vi "main(Test DQMH modules).vi"() -> ()   [LabVIEW 2018, in "Application.lvlib"] (continued)
      frame "Test DRV 27" {
        w4669 = 27  # DUT index(0-59)
        n2023 = disable-structure shown="LOGGING==TRUE" {
          disable-tunnel: w4670 -> [w4705 _]
          frame condition #0 (active) {
            n2024 = Empty String/Path?(string/path=w4705) -> (empty?=w4708:bool)
            n2025 = Select(t="Quece timeout", s=w4708, f=w4705) -> (s? t:f=w4704:string)
            n2026 = call "string log (SubVI).vi"("Enum"=enum16{"Init", "Log", "Read"}."Log", "state Name"=w4704) -> ()  [unwired: 8 in, 2 out]
          }
          frame condition #1 {
          }
        }
        n2027 = call "progress string(SubVI).vi"("String 3"=w4670, "String in"=w4671) -> ("String out"=w4672:string)  [unwired: 9 in]
        n2028 = call "FGV Driver Data.vi"("DUT index(1-60)"=w4669) -> ("DUT SC"=w4668:bool)  [unwired: 7 in, 3 out]
        n2029 = case shown="False" w4668 {
          tunnel: [w4697 _] -> w4677
          tunnel: w4674 -> [w4696 _]
          frame False {
            w4684 = T11 {"command"="", "command data"=variant} ("element")
            w4683 = "MEAS.mux6_1"
            n2030 = To Variant(anything=T4."mux6-1_channel0" ("mux6_1(3wires)_encode")) -> (Variant=w4682:variant)
            n2031 = To Variant(anything=T4."mux6_1_channel3_3" ("mux6_1(3wires)_encode")) -> (Variant=w4694:variant)
            n2032 = To Variant(anything=T4."mux6_1_channel3_2" ("mux6_1(3wires)_encode")) -> (Variant=w4692:variant)
            n2033 = Bundle By Name(cluster=w4684, "command"=w4683, "command data"=w4692) -> (w4691:T11)
            n2034 = Bundle By Name(cluster=w4684, "command"=w4683, "command data"=w4694) -> (w4690:T11)
            n2035 = Bundle By Name(cluster=w4684, "command"=w4683, "command data"=w4682) -> ()  [unwired: 1 out]
            n2036 = Bundle By Name(cluster=w4684, "command"="MEAS.DMM dual read") -> (w4688:T11)
            n2037 = Build Array(w4691, w4690, w4688) -> (w4686:T11[])
            n2038 = Reverse 1D Array(array=w4686) -> (reversed array=w4687:T11[])
            n2039 = for {
              tunnel: [w4703] -> w4697 mode=indexing
              tunnel: w4696 -> [w4702]
              tunnel: w4687 -> [w4701] mode=indexing
              n2040 = Unbundle By Name(w4701) -> ("command"=w4700:string, "command data"=w4699:variant)
              n2041 = call "App enquece.vi"("Priority Enquece"=TRUE, "command data"=w4699, "command"=w4700, "queue in"=w4702) -> ("error out"=w4703:errorcluster)  [unwired: 6 in, 1 out]
            }
          }
          frame True {
          }
        }
        n2042 = Merge Errors(w4675, w4677) -> (w4676:errorcluster)
      }
      frame "Test DRV 28" {
        w4710 = 28  # DUT index(0-59)
        n2043 = disable-structure shown="LOGGING==TRUE" {
          disable-tunnel: w4711 -> [w4746 _]
          frame condition #0 (active) {
            n2044 = Empty String/Path?(string/path=w4746) -> (empty?=w4749:bool)
            n2045 = Select(t="Quece timeout", s=w4749, f=w4746) -> (s? t:f=w4745:string)
            n2046 = call "string log (SubVI).vi"("Enum"=enum16{"Init", "Log", "Read"}."Log", "state Name"=w4745) -> ()  [unwired: 8 in, 2 out]
          }
          frame condition #1 {
          }
        }
        n2047 = call "progress string(SubVI).vi"("String 3"=w4711, "String in"=w4712) -> ("String out"=w4713:string)  [unwired: 9 in]
        n2048 = call "FGV Driver Data.vi"("DUT index(1-60)"=w4710) -> ("DUT SC"=w4709:bool)  [unwired: 7 in, 3 out]
        n2049 = case shown="False" w4709 {
          tunnel: [w4738 _] -> w4718
          tunnel: w4715 -> [w4737 _]
          frame False {
            w4723 = T11 {"command"="", "command data"=variant} ("element")
            w4725 = "MEAS.mux6_1"
            n2050 = To Variant(anything=T4."mux6-1_channel0" ("mux6_1(3wires)_encode")) -> (Variant=w4724:variant)
            n2051 = To Variant(anything=T4."mux6_1_channel4_3" ("mux6_1(3wires)_encode")) -> (Variant=w4735:variant)
            n2052 = To Variant(anything=T4."mux6_1_channel4_2" ("mux6_1(3wires)_encode")) -> (Variant=w4733:variant)
            n2053 = Bundle By Name(cluster=w4723, "command"=w4725, "command data"=w4733) -> (w4732:T11)
            n2054 = Bundle By Name(cluster=w4723, "command"=w4725, "command data"=w4735) -> (w4731:T11)
            n2055 = Bundle By Name(cluster=w4723, "command"=w4725, "command data"=w4724) -> ()  [unwired: 1 out]
            n2056 = Bundle By Name(cluster=w4723, "command"="MEAS.DMM dual read") -> (w4729:T11)
            n2057 = Build Array(w4732, w4731, w4729) -> (w4727:T11[])
            n2058 = Reverse 1D Array(array=w4727) -> (reversed array=w4728:T11[])
            n2059 = for {
              tunnel: [w4744] -> w4738 mode=indexing
              tunnel: w4737 -> [w4743]
              tunnel: w4728 -> [w4742] mode=indexing
              n2060 = Unbundle By Name(w4742) -> ("command"=w4741:string, "command data"=w4740:variant)
              n2061 = call "App enquece.vi"("Priority Enquece"=TRUE, "command data"=w4740, "command"=w4741, "queue in"=w4743) -> ("error out"=w4744:errorcluster)  [unwired: 6 in, 1 out]
            }
          }
          frame True {
          }
        }
        n2062 = Merge Errors(w4716, w4718) -> (w4717:errorcluster)
      }
      frame "Test DRV 29" {
        w4751 = 29  # DUT index(0-59)
        n2063 = disable-structure shown="LOGGING==TRUE" {
          disable-tunnel: w4752 -> [w4787 _]
          frame condition #0 (active) {
            n2064 = Empty String/Path?(string/path=w4787) -> (empty?=w4790:bool)
            n2065 = Select(t="Quece timeout", s=w4790, f=w4787) -> (s? t:f=w4786:string)
            n2066 = call "string log (SubVI).vi"("Enum"=enum16{"Init", "Log", "Read"}."Log", "state Name"=w4786) -> ()  [unwired: 8 in, 2 out]
          }
          frame condition #1 {
          }
        }
        n2067 = call "progress string(SubVI).vi"("String 3"=w4752, "String in"=w4753) -> ("String out"=w4754:string)  [unwired: 9 in]
        n2068 = call "FGV Driver Data.vi"("DUT index(1-60)"=w4751) -> ("DUT SC"=w4750:bool)  [unwired: 7 in, 3 out]
        n2069 = case shown="False" w4750 {
          tunnel: [w4779 _] -> w4759
          tunnel: w4756 -> [w4778 _]
          frame False {
            w4766 = T11 {"command"="", "command data"=variant} ("element")
            w4765 = "MEAS.mux6_1"
            n2070 = To Variant(anything=T4."mux6-1_channel0" ("mux6_1(3wires)_encode")) -> (Variant=w4764:variant)
            n2071 = To Variant(anything=T4."mux6_1_channel5_3" ("mux6_1(3wires)_encode")) -> (Variant=w4776:variant)
            n2072 = To Variant(anything=T4."mux6_1_channel5_2" ("mux6_1(3wires)_encode")) -> (Variant=w4774:variant)
            n2073 = Bundle By Name(cluster=w4766, "command"=w4765, "command data"=w4774) -> (w4773:T11)
            n2074 = Bundle By Name(cluster=w4766, "command"=w4765, "command data"=w4776) -> (w4772:T11)
            n2075 = Bundle By Name(cluster=w4766, "command"=w4765, "command data"=w4764) -> ()  [unwired: 1 out]
            n2076 = Bundle By Name(cluster=w4766, "command"="MEAS.DMM dual read") -> (w4770:T11)
            n2077 = Build Array(w4773, w4772, w4770) -> (w4768:T11[])
            n2078 = Reverse 1D Array(array=w4768) -> (reversed array=w4769:T11[])
            n2079 = for {
              tunnel: [w4785] -> w4779 mode=indexing
              tunnel: w4778 -> [w4784]
              tunnel: w4769 -> [w4783] mode=indexing
              n2080 = Unbundle By Name(w4783) -> ("command"=w4782:string, "command data"=w4781:variant)
              n2081 = call "App enquece.vi"("Priority Enquece"=TRUE, "command data"=w4781, "command"=w4782, "queue in"=w4784) -> ("error out"=w4785:errorcluster)  [unwired: 6 in, 1 out]
            }
          }
          frame True {
          }
        }
        n2082 = Merge Errors(w4757, w4759) -> (w4758:errorcluster)
      }
      frame "Test DRV 30" {
        w4791 = 30  # DUT index(0-59)
        n2083 = disable-structure shown="LOGGING==TRUE" {
          disable-tunnel: w4793 -> [w4828 _]
          frame condition #0 (active) {
            n2084 = Empty String/Path?(string/path=w4828) -> (empty?=w4831:bool)
            n2085 = Select(t="Quece timeout", s=w4831, f=w4828) -> (s? t:f=w4827:string)
            n2086 = call "string log (SubVI).vi"("Enum"=enum16{"Init", "Log", "Read"}."Log", "state Name"=w4827) -> ()  [unwired: 8 in, 2 out]
          }
          frame condition #1 {
          }
        }
        n2087 = call "progress string(SubVI).vi"("String 3"=w4793, "String in"=w4794) -> ("String out"=w4795:string)  [unwired: 9 in]
        n2088 = call "FGV Driver Data.vi"("DUT index(1-60)"=w4791) -> ("DUT SC"=w4792:bool)  [unwired: 7 in, 3 out]
        n2089 = case shown="False" w4792 {
          tunnel: [w4820 _] -> w4800
          tunnel: w4797 -> [w4819 _]
          frame False {
            w4807 = T11 {"command"="", "command data"=variant} ("element")
            w4806 = "MEAS.mux6_1"
            n2090 = To Variant(anything=T4."mux6-1_channel0" ("mux6_1(3wires)_encode")) -> (Variant=w4805:variant)
            n2091 = To Variant(anything=T4."mux6_1_channel6_3" ("mux6_1(3wires)_encode")) -> (Variant=w4817:variant)
            n2092 = To Variant(anything=T4."mux6_1_channel6_2" ("mux6_1(3wires)_encode")) -> (Variant=w4815:variant)
            n2093 = Bundle By Name(cluster=w4807, "command"=w4806, "command data"=w4815) -> (w4814:T11)
            n2094 = Bundle By Name(cluster=w4807, "command"=w4806, "command data"=w4817) -> (w4813:T11)
            n2095 = Bundle By Name(cluster=w4807, "command"=w4806, "command data"=w4805) -> ()  [unwired: 1 out]
            n2096 = Bundle By Name(cluster=w4807, "command"="MEAS.DMM dual read") -> (w4811:T11)
            n2097 = Build Array(w4814, w4813, w4811) -> (w4809:T11[])
            n2098 = Reverse 1D Array(array=w4809) -> (reversed array=w4810:T11[])
            n2099 = for {
              tunnel: [w4826] -> w4820 mode=indexing
              tunnel: w4819 -> [w4825]
              tunnel: w4810 -> [w4824] mode=indexing
              n2100 = Unbundle By Name(w4824) -> ("command"=w4823:string, "command data"=w4822:variant)
              n2101 = call "App enquece.vi"("Priority Enquece"=TRUE, "command data"=w4822, "command"=w4823, "queue in"=w4825) -> ("error out"=w4826:errorcluster)  [unwired: 6 in, 1 out]
            }
          }
          frame True {
          }
        }
        n2102 = Merge Errors(w4798, w4800) -> (w4799:errorcluster)
      }
      frame "Test DRV 31" {
        w4833 = 31  # DUT index(0-59)
        n2103 = disable-structure shown="LOGGING==TRUE" {
          disable-tunnel: w4834 -> [w4869 _]
          frame condition #0 (active) {
            n2104 = Empty String/Path?(string/path=w4869) -> (empty?=w4872:bool)
            n2105 = Select(t="Quece timeout", s=w4872, f=w4869) -> (s? t:f=w4868:string)
            n2106 = call "string log (SubVI).vi"("Enum"=enum16{"Init", "Log", "Read"}."Log", "state Name"=w4868) -> ()  [unwired: 8 in, 2 out]
          }
          frame condition #1 {
          }
        }
        n2107 = call "progress string(SubVI).vi"("String 3"=w4834, "String in"=w4835) -> ("String out"=w4836:string)  [unwired: 9 in]
        n2108 = call "FGV Driver Data.vi"("DUT index(1-60)"=w4833) -> ("DUT SC"=w4832:bool)  [unwired: 7 in, 3 out]
        n2109 = case shown="False" w4832 {
          tunnel: [w4861 _] -> w4841
          tunnel: w4838 -> [w4860 _]
          frame False {
            w4848 = T11 {"command"="", "command data"=variant} ("element")
            w4847 = "MEAS.mux6_1"
            n2110 = To Variant(anything=T4."mux6-1_channel0" ("mux6_1(3wires)_encode")) -> (Variant=w4846:variant)
            n2111 = To Variant(anything=T4."mux6_1_channel1_3" ("mux6_1(3wires)_encode")) -> (Variant=w4858:variant)
            n2112 = To Variant(anything=T4."mux6-1_channel1_2" ("mux6_1(3wires)_encode")) -> (Variant=w4856:variant)
            n2113 = Bundle By Name(cluster=w4848, "command"=w4847, "command data"=w4856) -> (w4855:T11)
            n2114 = Bundle By Name(cluster=w4848, "command"=w4847, "command data"=w4858) -> (w4854:T11)
            n2115 = Bundle By Name(cluster=w4848, "command"=w4847, "command data"=w4846) -> ()  [unwired: 1 out]
            n2116 = Bundle By Name(cluster=w4848, "command"="MEAS.DMM dual read") -> (w4852:T11)
            n2117 = Build Array(w4855, w4854, w4852) -> (w4850:T11[])
            n2118 = Reverse 1D Array(array=w4850) -> (reversed array=w4851:T11[])
            n2119 = for {
              tunnel: [w4867] -> w4861 mode=indexing
              tunnel: w4860 -> [w4866]
              tunnel: w4851 -> [w4865] mode=indexing
              n2120 = Unbundle By Name(w4865) -> ("command"=w4864:string, "command data"=w4863:variant)
              n2121 = call "App enquece.vi"("Priority Enquece"=TRUE, "command data"=w4863, "command"=w4864, "queue in"=w4866) -> ("error out"=w4867:errorcluster)  [unwired: 6 in, 1 out]
            }
          }
          frame True {
          }
        }
        n2122 = Merge Errors(w4839, w4841) -> (w4840:errorcluster)
      }
      frame "Test DRV 32" {
        w4874 = 32  # DUT index(0-59)
        n2123 = disable-structure shown="LOGGING==TRUE" {
          disable-tunnel: w4875 -> [w4910 _]
          frame condition #0 (active) {
            n2124 = Empty String/Path?(string/path=w4910) -> (empty?=w4913:bool)
            n2125 = Select(t="Quece timeout", s=w4913, f=w4910) -> (s? t:f=w4909:string)
            n2126 = call "string log (SubVI).vi"("Enum"=enum16{"Init", "Log", "Read"}."Log", "state Name"=w4909) -> ()  [unwired: 8 in, 2 out]
          }
          frame condition #1 {
          }
        }
        n2127 = call "progress string(SubVI).vi"("String 3"=w4875, "String in"=w4876) -> ("String out"=w4877:string)  [unwired: 9 in]
        n2128 = call "FGV Driver Data.vi"("DUT index(1-60)"=w4874) -> ("DUT SC"=w4873:bool)  [unwired: 7 in, 3 out]
        n2129 = case shown="False" w4873 {
          tunnel: [w4902 _] -> w4882
          tunnel: w4879 -> [w4901 _]
          frame False {
            w4889 = T11 {"command"="", "command data"=variant} ("element")
            w4888 = "MEAS.mux6_1"
            n2130 = To Variant(anything=T4."mux6-1_channel0" ("mux6_1(3wires)_encode")) -> (Variant=w4887:variant)
            n2131 = To Variant(anything=T4."mux6_1_channel2_3" ("mux6_1(3wires)_encode")) -> (Variant=w4899:variant)
            n2132 = To Variant(anything=T4."mux6_1_channel2_2" ("mux6_1(3wires)_encode")) -> (Variant=w4897:variant)
            n2133 = Bundle By Name(cluster=w4889, "command"=w4888, "command data"=w4897) -> (w4896:T11)
            n2134 = Bundle By Name(cluster=w4889, "command"=w4888, "command data"=w4899) -> (w4895:T11)
            n2135 = Bundle By Name(cluster=w4889, "command"=w4888, "command data"=w4887) -> ()  [unwired: 1 out]
            n2136 = Bundle By Name(cluster=w4889, "command"="MEAS.DMM dual read") -> (w4893:T11)
            n2137 = Build Array(w4896, w4895, w4893) -> (w4891:T11[])
            n2138 = Reverse 1D Array(array=w4891) -> (reversed array=w4892:T11[])
            n2139 = for {
              tunnel: [w4908] -> w4902 mode=indexing
              tunnel: w4901 -> [w4907]
              tunnel: w4892 -> [w4906] mode=indexing
              n2140 = Unbundle By Name(w4906) -> ("command"=w4905:string, "command data"=w4904:variant)
              n2141 = call "App enquece.vi"("Priority Enquece"=TRUE, "command data"=w4904, "command"=w4905, "queue in"=w4907) -> ("error out"=w4908:errorcluster)  [unwired: 6 in, 1 out]
            }
          }
          frame True {
          }
        }
        n2142 = Merge Errors(w4880, w4882) -> (w4881:errorcluster)
      }
      frame "Test DRV 33" {
        w4915 = 33  # DUT index(0-59)
        n2143 = disable-structure shown="LOGGING==TRUE" {
          disable-tunnel: w4916 -> [w4951 _]
          frame condition #0 (active) {
            n2144 = Empty String/Path?(string/path=w4951) -> (empty?=w4954:bool)
            n2145 = Select(t="Quece timeout", s=w4954, f=w4951) -> (s? t:f=w4950:string)
            n2146 = call "string log (SubVI).vi"("Enum"=enum16{"Init", "Log", "Read"}."Log", "state Name"=w4950) -> ()  [unwired: 8 in, 2 out]
          }
          frame condition #1 {
          }
        }
        n2147 = call "progress string(SubVI).vi"("String 3"=w4916, "String in"=w4917) -> ("String out"=w4918:string)  [unwired: 9 in]
        n2148 = call "FGV Driver Data.vi"("DUT index(1-60)"=w4915) -> ("DUT SC"=w4914:bool)  [unwired: 7 in, 3 out]
        n2149 = case shown="False" w4914 {
          tunnel: [w4943 _] -> w4923
          tunnel: w4920 -> [w4942 _]
          frame False {
            w4930 = T11 {"command"="", "command data"=variant} ("element")
            w4929 = "MEAS.mux6_1"
            n2150 = To Variant(anything=T4."mux6-1_channel0" ("mux6_1(3wires)_encode")) -> (Variant=w4928:variant)
            n2151 = To Variant(anything=T4."mux6_1_channel3_3" ("mux6_1(3wires)_encode")) -> (Variant=w4940:variant)
            n2152 = To Variant(anything=T4."mux6_1_channel3_2" ("mux6_1(3wires)_encode")) -> (Variant=w4938:variant)
            n2153 = Bundle By Name(cluster=w4930, "command"=w4929, "command data"=w4938) -> (w4937:T11)
            n2154 = Bundle By Name(cluster=w4930, "command"=w4929, "command data"=w4940) -> (w4936:T11)
            n2155 = Bundle By Name(cluster=w4930, "command"=w4929, "command data"=w4928) -> ()  [unwired: 1 out]
            n2156 = Bundle By Name(cluster=w4930, "command"="MEAS.DMM dual read") -> (w4934:T11)
            n2157 = Build Array(w4937, w4936, w4934) -> (w4932:T11[])
            n2158 = Reverse 1D Array(array=w4932) -> (reversed array=w4933:T11[])
            n2159 = for {
              tunnel: [w4949] -> w4943 mode=indexing
              tunnel: w4942 -> [w4948]
              tunnel: w4933 -> [w4947] mode=indexing
              n2160 = Unbundle By Name(w4947) -> ("command"=w4946:string, "command data"=w4945:variant)
              n2161 = call "App enquece.vi"("Priority Enquece"=TRUE, "command data"=w4945, "command"=w4946, "queue in"=w4948) -> ("error out"=w4949:errorcluster)  [unwired: 6 in, 1 out]
            }
          }
          frame True {
          }
        }
        n2162 = Merge Errors(w4921, w4923) -> (w4922:errorcluster)
      }
      frame "Test DRV 34" {
        w4956 = 34  # DUT index(0-59)
        n2163 = disable-structure shown="LOGGING==TRUE" {
          disable-tunnel: w4957 -> [w4992 _]
          frame condition #0 (active) {
            n2164 = Empty String/Path?(string/path=w4992) -> (empty?=w4995:bool)
            n2165 = Select(t="Quece timeout", s=w4995, f=w4992) -> (s? t:f=w4991:string)
            n2166 = call "string log (SubVI).vi"("Enum"=enum16{"Init", "Log", "Read"}."Log", "state Name"=w4991) -> ()  [unwired: 8 in, 2 out]
          }
          frame condition #1 {
          }
        }
        n2167 = call "progress string(SubVI).vi"("String 3"=w4957, "String in"=w4958) -> ("String out"=w4959:string)  [unwired: 9 in]
        n2168 = call "FGV Driver Data.vi"("DUT index(1-60)"=w4956) -> ("DUT SC"=w4955:bool)  [unwired: 7 in, 3 out]
        n2169 = case shown="False" w4955 {
          tunnel: [w4984 _] -> w4964
          tunnel: w4961 -> [w4983 _]
          frame False {
            w4971 = T11 {"command"="", "command data"=variant} ("element")
            w4970 = "MEAS.mux6_1"
            n2170 = To Variant(anything=T4."mux6-1_channel0" ("mux6_1(3wires)_encode")) -> (Variant=w4969:variant)
            n2171 = To Variant(anything=T4."mux6_1_channel4_3" ("mux6_1(3wires)_encode")) -> (Variant=w4981:variant)
            n2172 = To Variant(anything=T4."mux6_1_channel4_2" ("mux6_1(3wires)_encode")) -> (Variant=w4979:variant)
            n2173 = Bundle By Name(cluster=w4971, "command"=w4970, "command data"=w4979) -> (w4978:T11)
            n2174 = Bundle By Name(cluster=w4971, "command"=w4970, "command data"=w4981) -> (w4977:T11)
            n2175 = Bundle By Name(cluster=w4971, "command"=w4970, "command data"=w4969) -> ()  [unwired: 1 out]
            n2176 = Bundle By Name(cluster=w4971, "command"="MEAS.DMM dual read") -> (w4975:T11)
            n2177 = Build Array(w4978, w4977, w4975) -> (w4973:T11[])
            n2178 = Reverse 1D Array(array=w4973) -> (reversed array=w4974:T11[])
            n2179 = for {
              tunnel: [w4990] -> w4984 mode=indexing
              tunnel: w4983 -> [w4989]
              tunnel: w4974 -> [w4988] mode=indexing
              n2180 = Unbundle By Name(w4988) -> ("command"=w4987:string, "command data"=w4986:variant)
              n2181 = call "App enquece.vi"("Priority Enquece"=TRUE, "command data"=w4986, "command"=w4987, "queue in"=w4989) -> ("error out"=w4990:errorcluster)  [unwired: 6 in, 1 out]
            }
          }
          frame True {
          }
        }
        n2182 = Merge Errors(w4962, w4964) -> (w4963:errorcluster)
      }
      frame "Test DRV 35" {
        w4997 = 35  # DUT index(0-59)
        n2183 = disable-structure shown="LOGGING==TRUE" {
          disable-tunnel: w4998 -> [w5033 _]
          frame condition #0 (active) {
            n2184 = Empty String/Path?(string/path=w5033) -> (empty?=w5036:bool)
            n2185 = Select(t="Quece timeout", s=w5036, f=w5033) -> (s? t:f=w5032:string)
            n2186 = call "string log (SubVI).vi"("Enum"=enum16{"Init", "Log", "Read"}."Log", "state Name"=w5032) -> ()  [unwired: 8 in, 2 out]
          }
          frame condition #1 {
          }
        }
        n2187 = call "progress string(SubVI).vi"("String 3"=w4998, "String in"=w4999) -> ("String out"=w5000:string)  [unwired: 9 in]
        n2188 = call "FGV Driver Data.vi"("DUT index(1-60)"=w4997) -> ("DUT SC"=w4996:bool)  [unwired: 7 in, 3 out]
        n2189 = case shown="False" w4996 {
          tunnel: [w5025 _] -> w5005
          tunnel: w5002 -> [w5024 _]
          frame False {
            w5012 = T11 {"command"="", "command data"=variant} ("element")
            w5011 = "MEAS.mux6_1"
            n2190 = To Variant(anything=T4."mux6-1_channel0" ("mux6_1(3wires)_encode")) -> (Variant=w5010:variant)
            n2191 = To Variant(anything=T4."mux6_1_channel5_3" ("mux6_1(3wires)_encode")) -> (Variant=w5022:variant)
            n2192 = To Variant(anything=T4."mux6_1_channel5_2" ("mux6_1(3wires)_encode")) -> (Variant=w5020:variant)
            n2193 = Bundle By Name(cluster=w5012, "command"=w5011, "command data"=w5020) -> (w5019:T11)
            n2194 = Bundle By Name(cluster=w5012, "command"=w5011, "command data"=w5022) -> (w5018:T11)
            n2195 = Bundle By Name(cluster=w5012, "command"=w5011, "command data"=w5010) -> ()  [unwired: 1 out]
            n2196 = Bundle By Name(cluster=w5012, "command"="MEAS.DMM dual read") -> (w5016:T11)
            n2197 = Build Array(w5019, w5018, w5016) -> (w5014:T11[])
            n2198 = Reverse 1D Array(array=w5014) -> (reversed array=w5015:T11[])
            n2199 = for {
              tunnel: [w5031] -> w5025 mode=indexing
              tunnel: w5024 -> [w5030]
              tunnel: w5015 -> [w5029] mode=indexing
              n2200 = Unbundle By Name(w5029) -> ("command"=w5028:string, "command data"=w5027:variant)
              n2201 = call "App enquece.vi"("Priority Enquece"=TRUE, "command data"=w5027, "command"=w5028, "queue in"=w5030) -> ("error out"=w5031:errorcluster)  [unwired: 6 in, 1 out]
            }
          }
          frame True {
          }
        }
        n2202 = Merge Errors(w5003, w5005) -> (w5004:errorcluster)
      }
      frame "Test DRV 36" {
        w5038 = 36  # DUT index(0-59)
        n2203 = disable-structure shown="LOGGING==TRUE" {
          disable-tunnel: w5039 -> [w5074 _]
          frame condition #0 (active) {
            n2204 = Empty String/Path?(string/path=w5074) -> (empty?=w5077:bool)
            n2205 = Select(t="Quece timeout", s=w5077, f=w5074) -> (s? t:f=w5073:string)
            n2206 = call "string log (SubVI).vi"("Enum"=enum16{"Init", "Log", "Read"}."Log", "state Name"=w5073) -> ()  [unwired: 8 in, 2 out]
          }
          frame condition #1 {
          }
        }
        n2207 = call "progress string(SubVI).vi"("String 3"=w5039, "String in"=w5040) -> ("String out"=w5041:string)  [unwired: 9 in]
        n2208 = call "FGV Driver Data.vi"("DUT index(1-60)"=w5038) -> ("DUT SC"=w5037:bool)  [unwired: 7 in, 3 out]
        n2209 = case shown="False" w5037 {
          tunnel: [w5066 _] -> w5046
          tunnel: w5043 -> [w5065 _]
          frame False {
            w5053 = T11 {"command"="", "command data"=variant} ("element")
            w5052 = "MEAS.mux6_1"
            n2210 = To Variant(anything=T4."mux6-1_channel0" ("mux6_1(3wires)_encode")) -> (Variant=w5051:variant)
            n2211 = To Variant(anything=T4."mux6_1_channel6_3" ("mux6_1(3wires)_encode")) -> (Variant=w5063:variant)
            n2212 = To Variant(anything=T4."mux6_1_channel6_2" ("mux6_1(3wires)_encode")) -> (Variant=w5061:variant)
            n2213 = Bundle By Name(cluster=w5053, "command"=w5052, "command data"=w5061) -> (w5060:T11)
            n2214 = Bundle By Name(cluster=w5053, "command"=w5052, "command data"=w5063) -> (w5059:T11)
            n2215 = Bundle By Name(cluster=w5053, "command"=w5052, "command data"=w5051) -> ()  [unwired: 1 out]
            n2216 = Bundle By Name(cluster=w5053, "command"="MEAS.DMM dual read") -> (w5057:T11)
            n2217 = Build Array(w5060, w5059, w5057) -> (w5055:T11[])
            n2218 = Reverse 1D Array(array=w5055) -> (reversed array=w5056:T11[])
            n2219 = for {
              tunnel: [w5072] -> w5066 mode=indexing
              tunnel: w5065 -> [w5071]
              tunnel: w5056 -> [w5070] mode=indexing
              n2220 = Unbundle By Name(w5070) -> ("command"=w5069:string, "command data"=w5068:variant)
              n2221 = call "App enquece.vi"("Priority Enquece"=TRUE, "command data"=w5068, "command"=w5069, "queue in"=w5071) -> ("error out"=w5072:errorcluster)  [unwired: 6 in, 1 out]
            }
          }
          frame True {
          }
        }
        n2222 = Merge Errors(w5044, w5046) -> (w5045:errorcluster)
      }
      frame "Test DRV 37" {
        w5079 = 37  # DUT index(0-59)
        n2223 = disable-structure shown="LOGGING==TRUE" {
          disable-tunnel: w5080 -> [w5115 _]
          frame condition #0 (active) {
            n2224 = Empty String/Path?(string/path=w5115) -> (empty?=w5118:bool)
            n2225 = Select(t="Quece timeout", s=w5118, f=w5115) -> (s? t:f=w5114:string)
            n2226 = call "string log (SubVI).vi"("Enum"=enum16{"Init", "Log", "Read"}."Log", "state Name"=w5114) -> ()  [unwired: 8 in, 2 out]
          }
          frame condition #1 {
          }
        }
        n2227 = call "progress string(SubVI).vi"("String 3"=w5080, "String in"=w5081) -> ("String out"=w5082:string)  [unwired: 9 in]
        n2228 = call "FGV Driver Data.vi"("DUT index(1-60)"=w5079) -> ("DUT SC"=w5078:bool)  [unwired: 7 in, 3 out]
        n2229 = case shown="False" w5078 {
          tunnel: [w5107 _] -> w5087
          tunnel: w5084 -> [w5106 _]
          frame False {
            w5094 = T11 {"command"="", "command data"=variant} ("element")
            w5093 = "MEAS.mux6_1"
            n2230 = To Variant(anything=T4."mux6-1_channel0" ("mux6_1(3wires)_encode")) -> (Variant=w5092:variant)
            n2231 = To Variant(anything=T4."mux6_1_channel1_3" ("mux6_1(3wires)_encode")) -> (Variant=w5104:variant)
            n2232 = To Variant(anything=T4."mux6-1_channel1_2" ("mux6_1(3wires)_encode")) -> (Variant=w5102:variant)
            n2233 = Bundle By Name(cluster=w5094, "command"=w5093, "command data"=w5102) -> (w5101:T11)
            n2234 = Bundle By Name(cluster=w5094, "command"=w5093, "command data"=w5104) -> (w5100:T11)
            n2235 = Bundle By Name(cluster=w5094, "command"=w5093, "command data"=w5092) -> ()  [unwired: 1 out]
            n2236 = Bundle By Name(cluster=w5094, "command"="MEAS.DMM dual read") -> (w5098:T11)
            n2237 = Build Array(w5101, w5100, w5098) -> (w5096:T11[])
            n2238 = Reverse 1D Array(array=w5096) -> (reversed array=w5097:T11[])
            n2239 = for {
              tunnel: [w5113] -> w5107 mode=indexing
              tunnel: w5106 -> [w5112]
              tunnel: w5097 -> [w5111] mode=indexing
              n2240 = Unbundle By Name(w5111) -> ("command"=w5110:string, "command data"=w5109:variant)
              n2241 = call "App enquece.vi"("Priority Enquece"=TRUE, "command data"=w5109, "command"=w5110, "queue in"=w5112) -> ("error out"=w5113:errorcluster)  [unwired: 6 in, 1 out]
            }
          }
          frame True {
          }
        }
        n2242 = Merge Errors(w5085, w5087) -> (w5086:errorcluster)
      }
      frame "Test DRV 38" {
        w5120 = 38  # DUT index(0-59)
        n2243 = disable-structure shown="LOGGING==TRUE" {
          disable-tunnel: w5121 -> [w5156 _]
          frame condition #0 (active) {
            n2244 = Empty String/Path?(string/path=w5156) -> (empty?=w5159:bool)
            n2245 = Select(t="Quece timeout", s=w5159, f=w5156) -> (s? t:f=w5155:string)
            n2246 = call "string log (SubVI).vi"("Enum"=enum16{"Init", "Log", "Read"}."Log", "state Name"=w5155) -> ()  [unwired: 8 in, 2 out]
          }
          frame condition #1 {
          }
        }
        n2247 = call "progress string(SubVI).vi"("String 3"=w5121, "String in"=w5122) -> ("String out"=w5123:string)  [unwired: 9 in]
        n2248 = call "FGV Driver Data.vi"("DUT index(1-60)"=w5120) -> ("DUT SC"=w5119:bool)  [unwired: 7 in, 3 out]
        n2249 = case shown="False" w5119 {
          tunnel: [w5148 _] -> w5128
          tunnel: w5125 -> [w5147 _]
          frame False {
            w5135 = T11 {"command"="", "command data"=variant} ("element")
            w5134 = "MEAS.mux6_1"
            n2250 = To Variant(anything=T4."mux6-1_channel0" ("mux6_1(3wires)_encode")) -> (Variant=w5133:variant)
            n2251 = To Variant(anything=T4."mux6_1_channel2_3" ("mux6_1(3wires)_encode")) -> (Variant=w5145:variant)
            n2252 = To Variant(anything=T4."mux6_1_channel2_2" ("mux6_1(3wires)_encode")) -> (Variant=w5143:variant)
            n2253 = Bundle By Name(cluster=w5135, "command"=w5134, "command data"=w5143) -> (w5142:T11)
            n2254 = Bundle By Name(cluster=w5135, "command"=w5134, "command data"=w5145) -> (w5141:T11)
            n2255 = Bundle By Name(cluster=w5135, "command"=w5134, "command data"=w5133) -> ()  [unwired: 1 out]
            n2256 = Bundle By Name(cluster=w5135, "command"="MEAS.DMM dual read") -> (w5139:T11)
            n2257 = Build Array(w5142, w5141, w5139) -> (w5137:T11[])
            n2258 = Reverse 1D Array(array=w5137) -> (reversed array=w5138:T11[])
            n2259 = for {
              tunnel: [w5154] -> w5148 mode=indexing
              tunnel: w5147 -> [w5153]
              tunnel: w5138 -> [w5152] mode=indexing
              n2260 = Unbundle By Name(w5152) -> ("command"=w5151:string, "command data"=w5150:variant)
              n2261 = call "App enquece.vi"("Priority Enquece"=TRUE, "command data"=w5150, "command"=w5151, "queue in"=w5153) -> ("error out"=w5154:errorcluster)  [unwired: 6 in, 1 out]
            }
          }
          frame True {
          }
        }
        n2262 = Merge Errors(w5126, w5128) -> (w5127:errorcluster)
      }
      frame "Test DRV 39" {
        w5160 = 39  # DUT index(0-59)
        n2263 = disable-structure shown="LOGGING==TRUE" {
          disable-tunnel: w5162 -> [w5197 _]
          frame condition #0 (active) {
            n2264 = Empty String/Path?(string/path=w5197) -> (empty?=w5200:bool)
            n2265 = Select(t="Quece timeout", s=w5200, f=w5197) -> (s? t:f=w5196:string)
            n2266 = call "string log (SubVI).vi"("Enum"=enum16{"Init", "Log", "Read"}."Log", "state Name"=w5196) -> ()  [unwired: 8 in, 2 out]
          }
          frame condition #1 {
          }
        }
        n2267 = call "progress string(SubVI).vi"("String 3"=w5162, "String in"=w5163) -> ("String out"=w5164:string)  [unwired: 9 in]
        n2268 = call "FGV Driver Data.vi"("DUT index(1-60)"=w5160) -> ("DUT SC"=w5161:bool)  [unwired: 7 in, 3 out]
        n2269 = case shown="False" w5161 {
          tunnel: [w5189 _] -> w5169
          tunnel: w5166 -> [w5188 _]
          frame False {
            w5176 = T11 {"command"="", "command data"=variant} ("element")
            w5175 = "MEAS.mux6_1"
            n2270 = To Variant(anything=T4."mux6-1_channel0" ("mux6_1(3wires)_encode")) -> (Variant=w5174:variant)
            n2271 = To Variant(anything=T4."mux6_1_channel3_3" ("mux6_1(3wires)_encode")) -> (Variant=w5186:variant)
            n2272 = To Variant(anything=T4."mux6_1_channel3_2" ("mux6_1(3wires)_encode")) -> (Variant=w5184:variant)
            n2273 = Bundle By Name(cluster=w5176, "command"=w5175, "command data"=w5184) -> (w5183:T11)
            n2274 = Bundle By Name(cluster=w5176, "command"=w5175, "command data"=w5186) -> (w5182:T11)
            n2275 = Bundle By Name(cluster=w5176, "command"=w5175, "command data"=w5174) -> ()  [unwired: 1 out]
            n2276 = Bundle By Name(cluster=w5176, "command"="MEAS.DMM dual read") -> (w5180:T11)
            n2277 = Build Array(w5183, w5182, w5180) -> (w5178:T11[])
            n2278 = Reverse 1D Array(array=w5178) -> (reversed array=w5179:T11[])
            n2279 = for {
              tunnel: [w5195] -> w5189 mode=indexing
              tunnel: w5188 -> [w5194]
              tunnel: w5179 -> [w5193] mode=indexing
              n2280 = Unbundle By Name(w5193) -> ("command"=w5192:string, "command data"=w5191:variant)
              n2281 = call "App enquece.vi"("Priority Enquece"=TRUE, "command data"=w5191, "command"=w5192, "queue in"=w5194) -> ("error out"=w5195:errorcluster)  [unwired: 6 in, 1 out]
            }
          }
          frame True {
          }
        }
        n2282 = Merge Errors(w5167, w5169) -> (w5168:errorcluster)
      }
      frame "Test DRV 40" {
        w5202 = 40  # DUT index(0-59)
        n2283 = disable-structure shown="LOGGING==TRUE" {
          disable-tunnel: w5203 -> [w5238 _]
          frame condition #0 (active) {
            n2284 = Empty String/Path?(string/path=w5238) -> (empty?=w5241:bool)
            n2285 = Select(t="Quece timeout", s=w5241, f=w5238) -> (s? t:f=w5237:string)
            n2286 = call "string log (SubVI).vi"("Enum"=enum16{"Init", "Log", "Read"}."Log", "state Name"=w5237) -> ()  [unwired: 8 in, 2 out]
          }
          frame condition #1 {
          }
        }
        n2287 = call "progress string(SubVI).vi"("String 3"=w5203, "String in"=w5204) -> ("String out"=w5205:string)  [unwired: 9 in]
        n2288 = call "FGV Driver Data.vi"("DUT index(1-60)"=w5202) -> ("DUT SC"=w5201:bool)  [unwired: 7 in, 3 out]
        n2289 = case shown="False" w5201 {
          tunnel: [w5230 _] -> w5210
          tunnel: w5207 -> [w5229 _]
          frame False {
            w5217 = T11 {"command"="", "command data"=variant} ("element")
            w5216 = "MEAS.mux6_1"
            n2290 = To Variant(anything=T4."mux6-1_channel0" ("mux6_1(3wires)_encode")) -> (Variant=w5215:variant)
            n2291 = To Variant(anything=T4."mux6_1_channel4_3" ("mux6_1(3wires)_encode")) -> (Variant=w5227:variant)
            n2292 = To Variant(anything=T4."mux6_1_channel4_2" ("mux6_1(3wires)_encode")) -> (Variant=w5225:variant)
            n2293 = Bundle By Name(cluster=w5217, "command"=w5216, "command data"=w5225) -> (w5224:T11)
            n2294 = Bundle By Name(cluster=w5217, "command"=w5216, "command data"=w5227) -> (w5223:T11)
            n2295 = Bundle By Name(cluster=w5217, "command"=w5216, "command data"=w5215) -> ()  [unwired: 1 out]
            n2296 = Bundle By Name(cluster=w5217, "command"="MEAS.DMM dual read") -> (w5221:T11)
            n2297 = Build Array(w5224, w5223, w5221) -> (w5219:T11[])
            n2298 = Reverse 1D Array(array=w5219) -> (reversed array=w5220:T11[])
            n2299 = for {
              tunnel: [w5236] -> w5230 mode=indexing
              tunnel: w5229 -> [w5235]
              tunnel: w5220 -> [w5234] mode=indexing
              n2300 = Unbundle By Name(w5234) -> ("command"=w5233:string, "command data"=w5232:variant)
              n2301 = call "App enquece.vi"("Priority Enquece"=TRUE, "command data"=w5232, "command"=w5233, "queue in"=w5235) -> ("error out"=w5236:errorcluster)  [unwired: 6 in, 1 out]
            }
          }
          frame True {
          }
        }
        n2302 = Merge Errors(w5208, w5210) -> (w5209:errorcluster)
      }
      frame "Test DRV 41" {
        w5243 = 41  # DUT index(0-59)
        n2303 = disable-structure shown="LOGGING==TRUE" {
          disable-tunnel: w5244 -> [w5279 _]
          frame condition #0 (active) {
            n2304 = Empty String/Path?(string/path=w5279) -> (empty?=w5282:bool)
            n2305 = Select(t="Quece timeout", s=w5282, f=w5279) -> (s? t:f=w5278:string)
            n2306 = call "string log (SubVI).vi"("Enum"=enum16{"Init", "Log", "Read"}."Log", "state Name"=w5278) -> ()  [unwired: 8 in, 2 out]
          }
          frame condition #1 {
          }
        }
        n2307 = call "progress string(SubVI).vi"("String 3"=w5244, "String in"=w5245) -> ("String out"=w5246:string)  [unwired: 9 in]
        n2308 = call "FGV Driver Data.vi"("DUT index(1-60)"=w5243) -> ("DUT SC"=w5242:bool)  [unwired: 7 in, 3 out]
        n2309 = case shown="False" w5242 {
          tunnel: [w5271 _] -> w5251
          tunnel: w5248 -> [w5270 _]
          frame False {
            w5258 = T11 {"command"="", "command data"=variant} ("element")
            w5257 = "MEAS.mux6_1"
            n2310 = To Variant(anything=T4."mux6-1_channel0" ("mux6_1(3wires)_encode")) -> (Variant=w5256:variant)
            n2311 = To Variant(anything=T4."mux6_1_channel5_3" ("mux6_1(3wires)_encode")) -> (Variant=w5268:variant)
            n2312 = To Variant(anything=T4."mux6_1_channel5_2" ("mux6_1(3wires)_encode")) -> (Variant=w5266:variant)
            n2313 = Bundle By Name(cluster=w5258, "command"=w5257, "command data"=w5266) -> (w5265:T11)
            n2314 = Bundle By Name(cluster=w5258, "command"=w5257, "command data"=w5268) -> (w5264:T11)
            n2315 = Bundle By Name(cluster=w5258, "command"=w5257, "command data"=w5256) -> ()  [unwired: 1 out]
            n2316 = Bundle By Name(cluster=w5258, "command"="MEAS.DMM dual read") -> (w5262:T11)
            n2317 = Build Array(w5265, w5264, w5262) -> (w5260:T11[])
            n2318 = Reverse 1D Array(array=w5260) -> (reversed array=w5261:T11[])
            n2319 = for {
              tunnel: [w5277] -> w5271 mode=indexing
              tunnel: w5270 -> [w5276]
              tunnel: w5261 -> [w5275] mode=indexing
              n2320 = Unbundle By Name(w5275) -> ("command"=w5274:string, "command data"=w5273:variant)
              n2321 = call "App enquece.vi"("Priority Enquece"=TRUE, "command data"=w5273, "command"=w5274, "queue in"=w5276) -> ("error out"=w5277:errorcluster)  [unwired: 6 in, 1 out]
            }
          }
          frame True {
          }
        }
        n2322 = Merge Errors(w5249, w5251) -> (w5250:errorcluster)
      }
      frame "Test DRV 42" {
        w5284 = 42  # DUT index(0-59)
        n2323 = disable-structure shown="LOGGING==TRUE" {
          disable-tunnel: w5285 -> [w5320 _]
          frame condition #0 (active) {
            n2324 = Empty String/Path?(string/path=w5320) -> (empty?=w5323:bool)
            n2325 = Select(t="Quece timeout", s=w5323, f=w5320) -> (s? t:f=w5319:string)
            n2326 = call "string log (SubVI).vi"("Enum"=enum16{"Init", "Log", "Read"}."Log", "state Name"=w5319) -> ()  [unwired: 8 in, 2 out]
          }
          frame condition #1 {
          }
        }
        n2327 = call "progress string(SubVI).vi"("String 3"=w5285, "String in"=w5286) -> ("String out"=w5287:string)  [unwired: 9 in]
        n2328 = call "FGV Driver Data.vi"("DUT index(1-60)"=w5284) -> ("DUT SC"=w5283:bool)  [unwired: 7 in, 3 out]
        n2329 = case shown="False" w5283 {
          tunnel: [w5312 _] -> w5292
          tunnel: w5289 -> [w5311 _]
          frame False {
            w5299 = T11 {"command"="", "command data"=variant} ("element")
            w5298 = "MEAS.mux6_1"
            n2330 = To Variant(anything=T4."mux6-1_channel0" ("mux6_1(3wires)_encode")) -> (Variant=w5297:variant)
            n2331 = To Variant(anything=T4."mux6_1_channel6_3" ("mux6_1(3wires)_encode")) -> (Variant=w5309:variant)
            n2332 = To Variant(anything=T4."mux6_1_channel6_2" ("mux6_1(3wires)_encode")) -> (Variant=w5307:variant)
            n2333 = Bundle By Name(cluster=w5299, "command"=w5298, "command data"=w5307) -> (w5306:T11)
            n2334 = Bundle By Name(cluster=w5299, "command"=w5298, "command data"=w5309) -> (w5305:T11)
            n2335 = Bundle By Name(cluster=w5299, "command"=w5298, "command data"=w5297) -> ()  [unwired: 1 out]
            n2336 = Bundle By Name(cluster=w5299, "command"="MEAS.DMM dual read") -> (w5303:T11)
            n2337 = Build Array(w5306, w5305, w5303) -> (w5301:T11[])
            n2338 = Reverse 1D Array(array=w5301) -> (reversed array=w5302:T11[])
            n2339 = for {
              tunnel: [w5318] -> w5312 mode=indexing
              tunnel: w5311 -> [w5317]
              tunnel: w5302 -> [w5316] mode=indexing
              n2340 = Unbundle By Name(w5316) -> ("command"=w5315:string, "command data"=w5314:variant)
              n2341 = call "App enquece.vi"("Priority Enquece"=TRUE, "command data"=w5314, "command"=w5315, "queue in"=w5317) -> ("error out"=w5318:errorcluster)  [unwired: 6 in, 1 out]
            }
          }
          frame True {
          }
        }
        n2342 = Merge Errors(w5290, w5292) -> (w5291:errorcluster)
      }
      frame "Test DRV 43" {
        w5325 = 43  # DUT index(0-59)
        n2343 = disable-structure shown="LOGGING==TRUE" {
          disable-tunnel: w5326 -> [w5361 _]
          frame condition #0 (active) {
            n2344 = Empty String/Path?(string/path=w5361) -> (empty?=w5364:bool)
            n2345 = Select(t="Quece timeout", s=w5364, f=w5361) -> (s? t:f=w5360:string)
            n2346 = call "string log (SubVI).vi"("Enum"=enum16{"Init", "Log", "Read"}."Log", "state Name"=w5360) -> ()  [unwired: 8 in, 2 out]
          }
          frame condition #1 {
          }
        }
        n2347 = call "progress string(SubVI).vi"("String 3"=w5326, "String in"=w5327) -> ("String out"=w5328:string)  [unwired: 9 in]
        n2348 = call "FGV Driver Data.vi"("DUT index(1-60)"=w5325) -> ("DUT SC"=w5324:bool)  [unwired: 7 in, 3 out]
        n2349 = case shown="False" w5324 {
          tunnel: [w5353 _] -> w5333
          tunnel: w5330 -> [w5352 _]
          frame False {
            w5340 = T11 {"command"="", "command data"=variant} ("element")
            w5339 = "MEAS.mux6_1"
            n2350 = To Variant(anything=T4."mux6-1_channel0" ("mux6_1(3wires)_encode")) -> (Variant=w5338:variant)
            n2351 = To Variant(anything=T4."mux6_1_channel1_3" ("mux6_1(3wires)_encode")) -> (Variant=w5350:variant)
            n2352 = To Variant(anything=T4."mux6-1_channel1_2" ("mux6_1(3wires)_encode")) -> (Variant=w5348:variant)
            n2353 = Bundle By Name(cluster=w5340, "command"=w5339, "command data"=w5348) -> (w5347:T11)
            n2354 = Bundle By Name(cluster=w5340, "command"=w5339, "command data"=w5350) -> (w5346:T11)
            n2355 = Bundle By Name(cluster=w5340, "command"=w5339, "command data"=w5338) -> ()  [unwired: 1 out]
            n2356 = Bundle By Name(cluster=w5340, "command"="MEAS.DMM dual read") -> (w5344:T11)
            n2357 = Build Array(w5347, w5346, w5344) -> (w5342:T11[])
            n2358 = Reverse 1D Array(array=w5342) -> (reversed array=w5343:T11[])
            n2359 = for {
              tunnel: [w5359] -> w5353 mode=indexing
              tunnel: w5352 -> [w5358]
              tunnel: w5343 -> [w5357] mode=indexing
              n2360 = Unbundle By Name(w5357) -> ("command"=w5356:string, "command data"=w5355:variant)
              n2361 = call "App enquece.vi"("Priority Enquece"=TRUE, "command data"=w5355, "command"=w5356, "queue in"=w5358) -> ("error out"=w5359:errorcluster)  [unwired: 6 in, 1 out]
            }
          }
          frame True {
          }
        }
        n2362 = Merge Errors(w5331, w5333) -> (w5332:errorcluster)
      }
      frame "Test DRV 44" {
        w5366 = 44  # DUT index(0-59)
        n2363 = disable-structure shown="LOGGING==TRUE" {
          disable-tunnel: w5367 -> [w5402 _]
          frame condition #0 (active) {
            n2364 = Empty String/Path?(string/path=w5402) -> (empty?=w5405:bool)
            n2365 = Select(t="Quece timeout", s=w5405, f=w5402) -> (s? t:f=w5401:string)
            n2366 = call "string log (SubVI).vi"("Enum"=enum16{"Init", "Log", "Read"}."Log", "state Name"=w5401) -> ()  [unwired: 8 in, 2 out]
          }
          frame condition #1 {
          }
        }
        n2367 = call "progress string(SubVI).vi"("String 3"=w5367, "String in"=w5368) -> ("String out"=w5369:string)  [unwired: 9 in]
        n2368 = call "FGV Driver Data.vi"("DUT index(1-60)"=w5366) -> ("DUT SC"=w5365:bool)  [unwired: 7 in, 3 out]
        n2369 = case shown="False" w5365 {
          tunnel: [w5394 _] -> w5374
          tunnel: w5371 -> [w5393 _]
          frame False {
            w5381 = T11 {"command"="", "command data"=variant} ("element")
            w5380 = "MEAS.mux6_1"
            n2370 = To Variant(anything=T4."mux6-1_channel0" ("mux6_1(3wires)_encode")) -> (Variant=w5379:variant)
            n2371 = To Variant(anything=T4."mux6_1_channel2_3" ("mux6_1(3wires)_encode")) -> (Variant=w5391:variant)
            n2372 = To Variant(anything=T4."mux6_1_channel2_2" ("mux6_1(3wires)_encode")) -> (Variant=w5389:variant)
            n2373 = Bundle By Name(cluster=w5381, "command"=w5380, "command data"=w5389) -> (w5388:T11)
            n2374 = Bundle By Name(cluster=w5381, "command"=w5380, "command data"=w5391) -> (w5387:T11)
            n2375 = Bundle By Name(cluster=w5381, "command"=w5380, "command data"=w5379) -> ()  [unwired: 1 out]
            n2376 = Bundle By Name(cluster=w5381, "command"="MEAS.DMM dual read") -> (w5385:T11)
            n2377 = Build Array(w5388, w5387, w5385) -> (w5383:T11[])
            n2378 = Reverse 1D Array(array=w5383) -> (reversed array=w5384:T11[])
            n2379 = for {
              tunnel: [w5400] -> w5394 mode=indexing
              tunnel: w5393 -> [w5399]
              tunnel: w5384 -> [w5398] mode=indexing
              n2380 = Unbundle By Name(w5398) -> ("command"=w5397:string, "command data"=w5396:variant)
              n2381 = call "App enquece.vi"("Priority Enquece"=TRUE, "command data"=w5396, "command"=w5397, "queue in"=w5399) -> ("error out"=w5400:errorcluster)  [unwired: 6 in, 1 out]
            }
          }
          frame True {
          }
        }
        n2382 = Merge Errors(w5372, w5374) -> (w5373:errorcluster)
      }
      frame "Test DRV 45" {
        w5406 = 45  # DUT index(1-60)
        n2383 = disable-structure shown="LOGGING==TRUE" {
          disable-tunnel: w5408 -> [w5443 _]
          frame condition #0 (active) {
            n2384 = Empty String/Path?(string/path=w5443) -> (empty?=w5446:bool)
            n2385 = Select(t="Quece timeout", s=w5446, f=w5443) -> (s? t:f=w5442:string)
            n2386 = call "string log (SubVI).vi"("Enum"=enum16{"Init", "Log", "Read"}."Log", "state Name"=w5442) -> ()  [unwired: 8 in, 2 out]
          }
          frame condition #1 {
          }
        }
        n2387 = call "progress string(SubVI).vi"("String 3"=w5408, "String in"=w5409) -> ("String out"=w5410:string)  [unwired: 9 in]
        n2388 = call "FGV Driver Data.vi"("DUT index(1-60)"=w5406) -> ("DUT SC"=w5407:bool)  [unwired: 7 in, 3 out]
        n2389 = case shown="False" w5407 {
          tunnel: [w5435 _] -> w5415
          tunnel: w5412 -> [w5434 _]
          frame False {
            w5422 = T11 {"command"="", "command data"=variant} ("element")
            w5421 = "MEAS.mux6_1"
            n2390 = To Variant(anything=T4."mux6-1_channel0" ("mux6_1(3wires)_encode")) -> (Variant=w5420:variant)
            n2391 = To Variant(anything=T4."mux6_1_channel3_3" ("mux6_1(3wires)_encode")) -> (Variant=w5432:variant)
            n2392 = To Variant(anything=T4."mux6_1_channel3_2" ("mux6_1(3wires)_encode")) -> (Variant=w5430:variant)
            n2393 = Bundle By Name(cluster=w5422, "command"=w5421, "command data"=w5430) -> (w5429:T11)
            n2394 = Bundle By Name(cluster=w5422, "command"=w5421, "command data"=w5432) -> (w5428:T11)
            n2395 = Bundle By Name(cluster=w5422, "command"=w5421, "command data"=w5420) -> ()  [unwired: 1 out]
            n2396 = Bundle By Name(cluster=w5422, "command"="MEAS.DMM dual read") -> (w5426:T11)
            n2397 = Build Array(w5429, w5428, w5426) -> (w5424:T11[])
            n2398 = Reverse 1D Array(array=w5424) -> (reversed array=w5425:T11[])
            n2399 = for {
              tunnel: [w5441] -> w5435 mode=indexing
              tunnel: w5434 -> [w5440]
              tunnel: w5425 -> [w5439] mode=indexing
              n2400 = Unbundle By Name(w5439) -> ("command"=w5438:string, "command data"=w5437:variant)
              n2401 = call "App enquece.vi"("Priority Enquece"=TRUE, "command data"=w5437, "command"=w5438, "queue in"=w5440) -> ("error out"=w5441:errorcluster)  [unwired: 6 in, 1 out]
            }
          }
          frame True {
          }
        }
        n2402 = Merge Errors(w5413, w5415) -> (w5414:errorcluster)
      }
      frame "Test DRV 46" {
        w5448 = 46  # DUT index(0-59)
        n2403 = disable-structure shown="LOGGING==TRUE" {
          disable-tunnel: w5449 -> [w5484 _]
          frame condition #0 (active) {
            n2404 = Empty String/Path?(string/path=w5484) -> (empty?=w5487:bool)
            n2405 = Select(t="Quece timeout", s=w5487, f=w5484) -> (s? t:f=w5483:string)
            n2406 = call "string log (SubVI).vi"("Enum"=enum16{"Init", "Log", "Read"}."Log", "state Name"=w5483) -> ()  [unwired: 8 in, 2 out]
          }
          frame condition #1 {
          }
        }
        n2407 = call "progress string(SubVI).vi"("String 3"=w5449, "String in"=w5450) -> ("String out"=w5451:string)  [unwired: 9 in]
        n2408 = call "FGV Driver Data.vi"("DUT index(1-60)"=w5448) -> ("DUT SC"=w5447:bool)  [unwired: 7 in, 3 out]
        n2409 = case shown="False" w5447 {
          tunnel: [w5476 _] -> w5456
          tunnel: w5453 -> [w5475 _]
          frame False {
            w5463 = T11 {"command"="", "command data"=variant} ("element")
            w5462 = "MEAS.mux6_1"
            n2410 = To Variant(anything=T4."mux6-1_channel0" ("mux6_1(3wires)_encode")) -> (Variant=w5461:variant)
            n2411 = To Variant(anything=T4."mux6_1_channel4_3" ("mux6_1(3wires)_encode")) -> (Variant=w5473:variant)
            n2412 = To Variant(anything=T4."mux6_1_channel4_2" ("mux6_1(3wires)_encode")) -> (Variant=w5471:variant)
            n2413 = Bundle By Name(cluster=w5463, "command"=w5462, "command data"=w5471) -> (w5470:T11)
            n2414 = Bundle By Name(cluster=w5463, "command"=w5462, "command data"=w5473) -> (w5469:T11)
            n2415 = Bundle By Name(cluster=w5463, "command"=w5462, "command data"=w5461) -> ()  [unwired: 1 out]
            n2416 = Bundle By Name(cluster=w5463, "command"="MEAS.DMM dual read") -> (w5467:T11)
            n2417 = Build Array(w5470, w5469, w5467) -> (w5465:T11[])
            n2418 = Reverse 1D Array(array=w5465) -> (reversed array=w5466:T11[])
            n2419 = for {
              tunnel: [w5482] -> w5476 mode=indexing
              tunnel: w5475 -> [w5481]
              tunnel: w5466 -> [w5480] mode=indexing
              n2420 = Unbundle By Name(w5480) -> ("command"=w5479:string, "command data"=w5478:variant)
